vi "Spätzle_Control_myRIO.vi"(6 "error in":errorcluster) -> (0 "error out 2":errorcluster)   [LabVIEW 2014]
doc: "Mit diesem VI wird eine Autowäsche simuliert. Mit den Waschprogrammelementen wählen Sie die gewünschten Optionen aus. Wenn keine Option ausgewählt wird, ist die Hochdruckreinigung das Standardwaschprogramm. Nach Klick auf \"Start\" beginnt die Wäsche. Mit dem Element \"Schieberegler für Fahrzeugposition\" wird die Position des Fahrzeugs simuliert. Wenn sich das Fahrzeug in der falschen Position für das aktuelle Programm befindet, leuchtet die entsprechende Anzeige und das Fahrzeug muss bewegt werden. Die Anzeige der Waschanlage stellt den aktuellen Status des Waschprogramms dar. Mit der Schaltfläche \"Programm stoppen\" wird die Autowaschanlage sofort gestoppt."
uses:
  Controls/Indicators.ctl
  Controls/State Control Enum.ctl
  Controls/Conveyor Belt Functions.ctl
  <vilib>/myRIO/Instrument Drivers/Onboard IO/DIO/typedefs/DIO Reference.ctl
  <vilib>/myRIO/Common/Instrument Driver Framework/Utilities/typedefs/myRIO Generic Hardware Reference.ctl
  <vilib>/myRIO/Common/Instrument Driver Framework/Utilities/typedefs/Hardware Version Enum.ctl
  <vilib>/myRIO/Common/Instrument Driver Framework/Utilities/typedefs/myRIO v1.0 Reference.ctl
  <vilib>/myRIO/Common/Instrument Driver Framework/Utilities/typedefs/Generic FPGA Reference.ctl
  <vilib>/myRIO/Common/Instrument Driver Framework/myRIO v1.0/DIO/typedefs/DIO Channels List.ctl
  <vilib>/myRIO/Common/Instrument Driver Framework/myRIO v1.0/DIO/typedefs/DIO Channels Enum.ctl
  <vilib>/userdefined/High Color/nirio_resource_hc.ctl
  <vilib>/myRIO/Common/Instrument Driver Framework/myRIO v1.0/DIO/vis/myRIO v1.1 Open DIO.vi
  <vilib>/myRIO/Common/Instrument Driver Framework/Utilities/vis/Is FPGA Ref Available.vi
  <vilib>/myRIO/Instrument Drivers/Onboard IO/DIO/vis/Write.vi
  <vilib>/myRIO/Common/Instrument Driver Framework/Utilities/vis/Validate Channels.vi
  <vilib>/myRIO/Common/Instrument Driver Framework/myRIO v1.0/DIO/vis/myRIO v1.0 Reserve DIO.vi
  <vilib>/myRIO/Common/Instrument Driver Framework/myRIO v1.0/DIO/vis/myRIO v1.0 Close DIO.vi
  <vilib>/myRIO/Common/Instrument Driver Framework/myRIO v1.0/UART/vis/myRIO v1.0 Close UART.vi
  <vilib>/myRIO/Common/Instrument Driver Framework/myRIO v1.0/Resource Manager/vis/myRIO v1.0 Reserve Channel List.vi
  <vilib>/myRIO/Common/Instrument Driver Framework/myRIO v1.0/DIO/vis/myRIO v1.0 Build MUX Configuration DIO.vi
  <vilib>/myRIO/Common/Instrument Driver Framework/myRIO v1.0/DIO/vis/myRIO v1.0 Unreserve DIO.vi
  <vilib>/myRIO/Common/Instrument Driver Framework/myRIO v1.0/Resource Manager/vis/myRIO v1.0 Reserve Channel.vi
  <vilib>/myRIO/Common/Instrument Driver Framework/myRIO v1.0/Resource Manager/vis/myRIO v1.0 Unreserve Channel.vi
  <vilib>/myRIO/Common/Instrument Driver Framework/myRIO v1.0/Resource Manager/vis/myRIO v1.0 Create Configuration List.vi
  <vilib>/myRIO/Common/Instrument Driver Framework/myRIO v1.0/Resource Manager/vis/myRIO v1.0 Unreserve Channel List.vi
  <vilib>/myRIO/Common/Instrument Driver Framework/myRIO v1.0/Resource Manager/vis/myRIO v1.0 Build Mutex Name.vi
  <vilib>/Utility/VariantDataType/GetNumericInfo.vi
  <vilib>/Utility/error.llb/Error Cluster From Error Code.vi
  <vilib>/myRIO/Common/Instrument Driver Framework/myRIO v1.0/myRIO v1.1 Open.vi
  <vilib>/myRIO/Common/Instrument Driver Framework/Utilities/vis/IO Manager.vi
  <vilib>/myRIO/Common/Instrument Driver Framework/Utilities/vis/Configuration Manager.vi
  <vilib>/myRIO/Common/Instrument Driver Framework/myRIO v1.0/Resource Manager/vis/myRIO v1.0 Configure IO.vi
  <vilib>/myRIO/Common/Instrument Driver Framework/myRIO v1.0/myRIO v1.0 Close.vi
  <vilib>/myRIO/Common/Instrument Driver Framework/myRIO v1.0/DIO/vis/myRIO v1.0 Read DIO.vi
  <vilib>/myRIO/Common/Instrument Driver Framework/myRIO v1.0/DIO/vis/myRIO v1.0 Write DIO.vi
  <vilib>/myRIO/Common/Instrument Driver Framework/myRIO v1.0/DIO/vis/myRIO v1.0 Shutdown DIO.vi
  <vilib>/myRIO/Common/Instrument Driver Framework/Utilities/vis/FPGA Ref Manager.vi
  <vilib>/myRIO/Common/Instrument Driver Framework/myRIO v1.0/myRIO v1.0 Reset FPGA.vi
  <vilib>/myRIO/Common/Instrument Driver Framework/myRIO v1.0/IRQ/vis/myRIO v1.0 IRQ Info FGV.vi
  <vilib>/myRIO/Common/Instrument Driver Framework/myRIO v1.0/IRQ/vis/myRIO v1.0 Timer IRQ Info FGV.vi
  <vilib>/myRIO/Common/Instrument Driver Framework/myRIO v1.0/IRQ/vis/myRIO v1.0 ISR Agent.vi
  <vilib>/myRIO/Instrument Drivers/Onboard IO/DIO/vis/myRIO DIO Open.xnode
  <vilib>/myRIO/Express VI/Onboard IO/DO/DO Express VI.xnode
  <vilib>/myRIO/Instrument Drivers/Onboard IO/DIO/DIO.lvlib
  <vilib>/myRIO/Instrument Drivers/Utilities/Utilities.lvlib
panel:
  in  "stop":bool
  out "?":T1
  out "Busy":bool
  # "Machine Status"
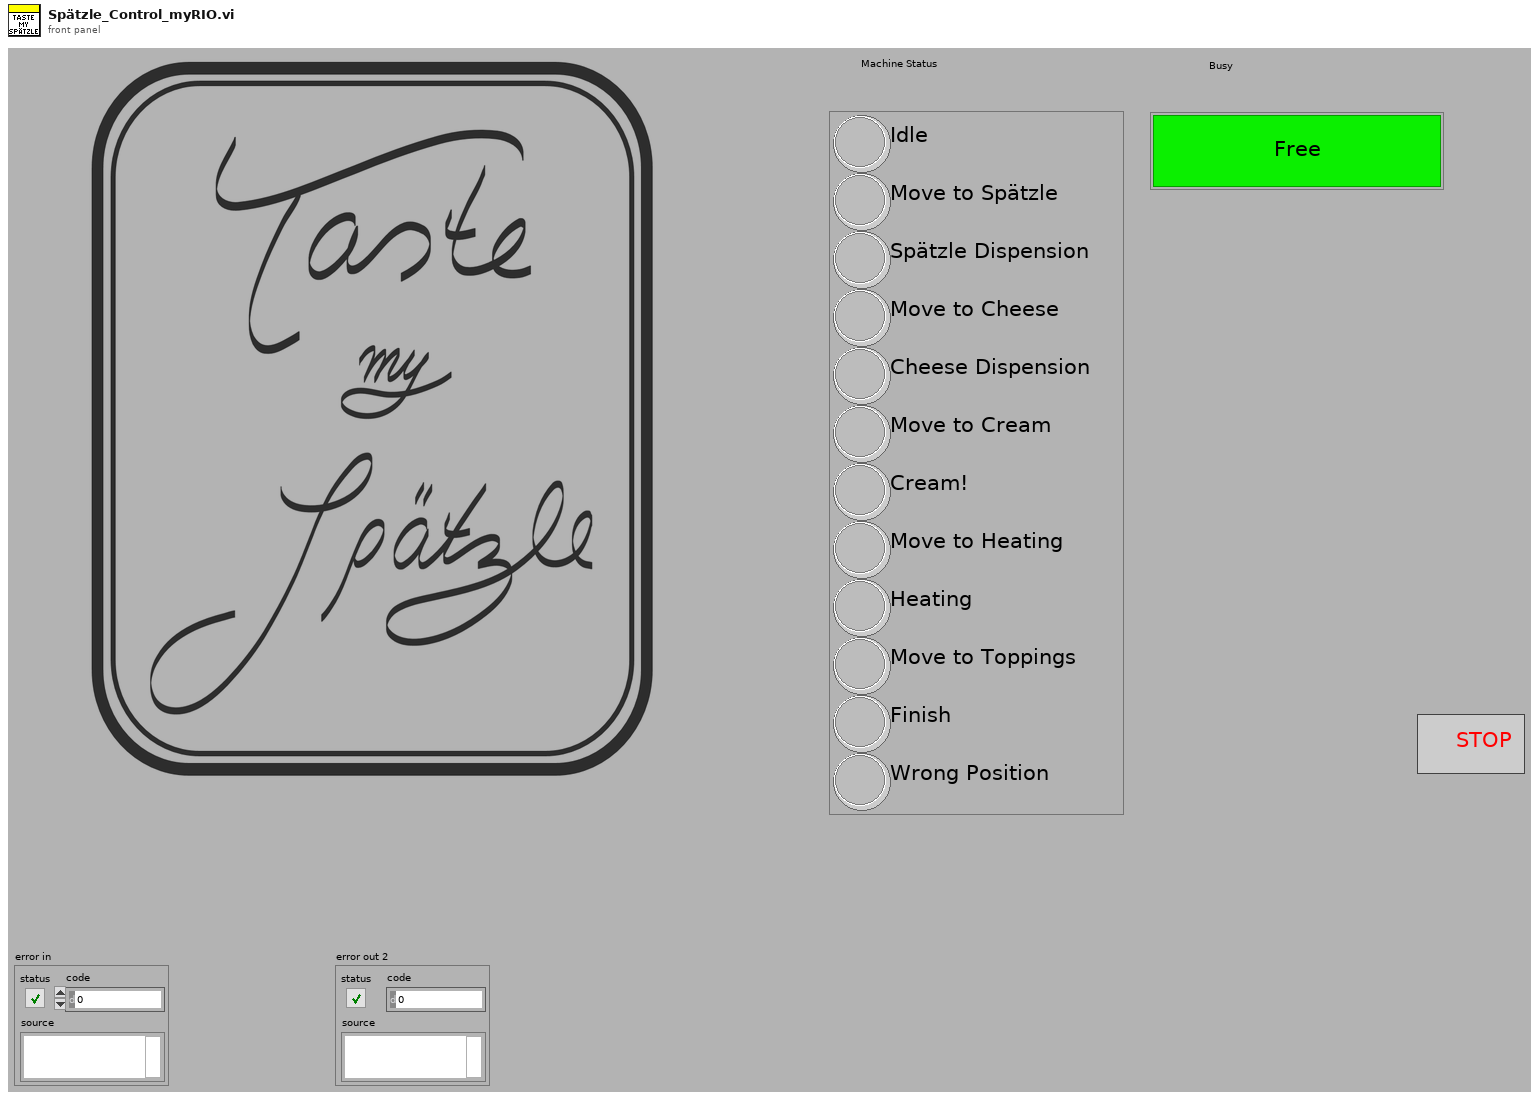
[diagram p1: front panel]
types:
  T1 = typedef "Indicators.ctl" = cluster{"Idle":bool, "Move to Spätzle":bool, "Spätzle Dispension":bool, "Move to Cheese":bool, "Cheese Dispension":bool, "Move to Cream":bool, "Cream!":bool, "Move to Heating":bool, "Heating":bool, "Move to Toppings":bool, "Finish":bool, "Wrong Position":bool}
  T2 = typedef "Conveyor Belt Functions.ctl" = enum16{"Move Forward", "Move Backward", "Stop"}
  T3 = typedef "State Control Enum.ctl" = enum16{"Initialize", "Wait for Start", "Plate Dispension", "Spätzle Dispension", "Move to Cream", "Cream", "Move to Heating", "Heating", "Cheese Dispension", "Onion Dispension", "Garlic Dispension", "Butter Dispension", "Move to Spätzle", "Move To Cheese", "Move to Exit", "Stop", "Skip"}
  T4 = typedef "DIO.lvlib/DIO Reference.ctl" = cluster{"myRIO Reference":T5, "DIO Channels List":T9}
  T5 = typedef "myRIO Generic Hardware Reference.ctl" = cluster{"myRIO Model":T6, "myRIO Hardware Reference":T7}
  T6 = typedef "Hardware Version Enum.ctl" = enum16{"Unknown", "myRIO-1900", "myRIO-1950"}
  T7 = typedef "myRIO v1.0 Reference.ctl" = cluster{"Generic FPGA Reference":T8, "Allow multiple opens":bool}
  T8 = typedef "Generic FPGA Reference.ctl" = refnum<k20>
  T9 = typedef "DIO Channels List.ctl" = T10[]
  T10 = typedef "DIO Channels Enum.ctl" = enum16{"Not Connected", "C/DIO0", "C/DIO1", "C/DIO2", "C/DIO3", "C/DIO4", "C/DIO5", "C/DIO6", "C/DIO7", "A/DIO0", "A/DIO1", "A/DIO2", "A/DIO3", "A/DIO4", "A/DIO5", "A/DIO6", "A/DIO7", "A/DIO8", "A/DIO9", "A/DIO10", "A/DIO11", "A/DIO12", "A/DIO13", "A/DIO14", "A/DIO15", "B/DIO0", "B/DIO1", "B/DIO2", "B/DIO3", "B/DIO4", "B/DIO5", "B/DIO6", "B/DIO7", "B/DIO8", "B/DIO9", "B/DIO10", "B/DIO11", "B/DIO12", "B/DIO13", "B/DIO14", "B/DIO15", "LED0", "LED1", "LED2", "LED3", "Button0"}
  T11 = typedef "nirio_resource_hc.ctl" = tag
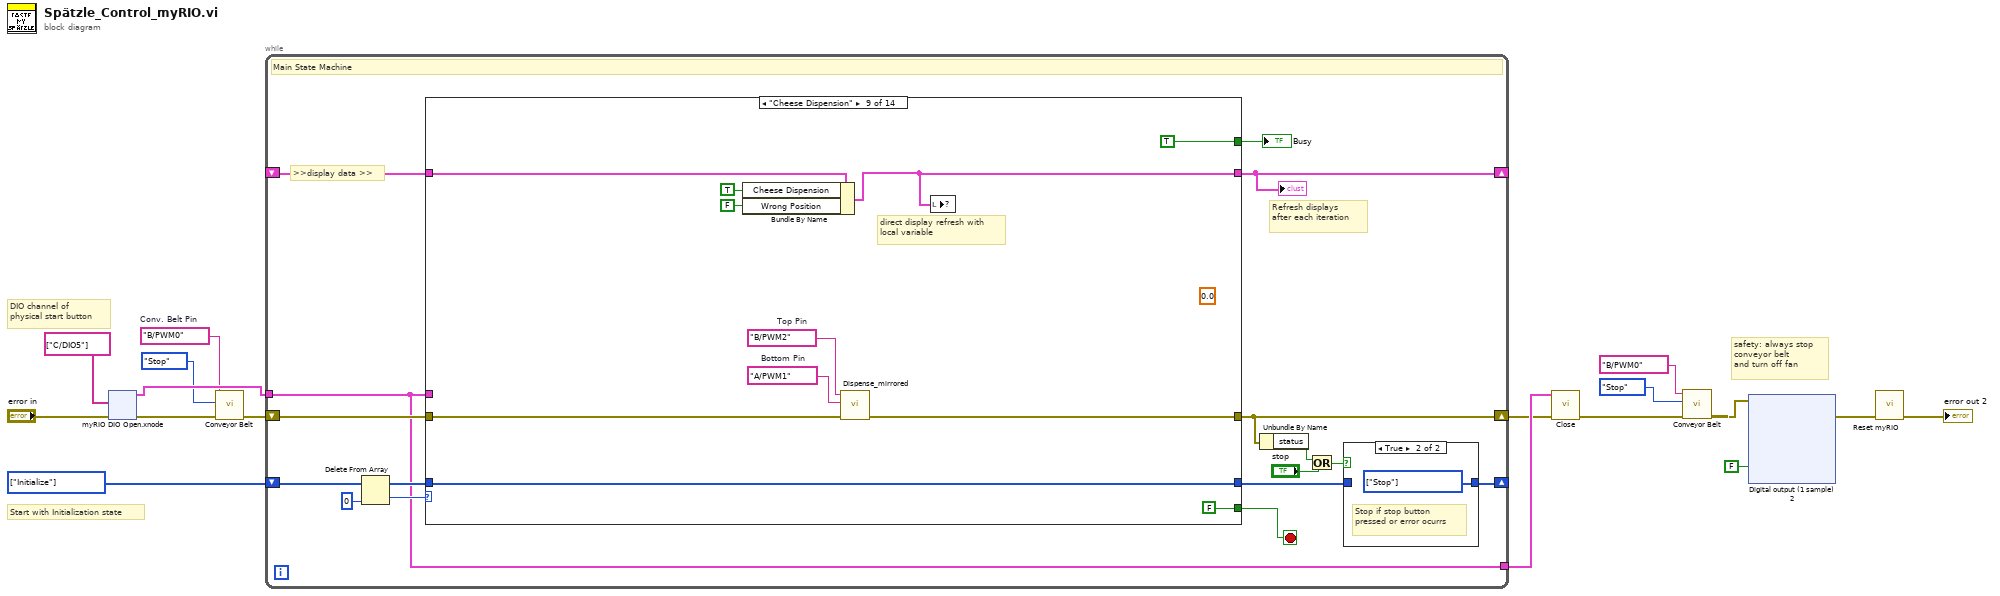
[diagram p0: block diagram]
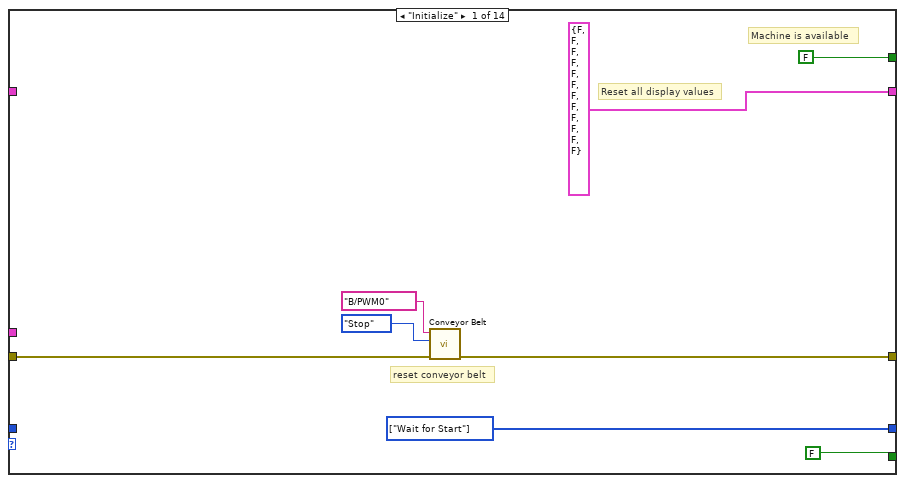
[diagram p3: hidden frame]
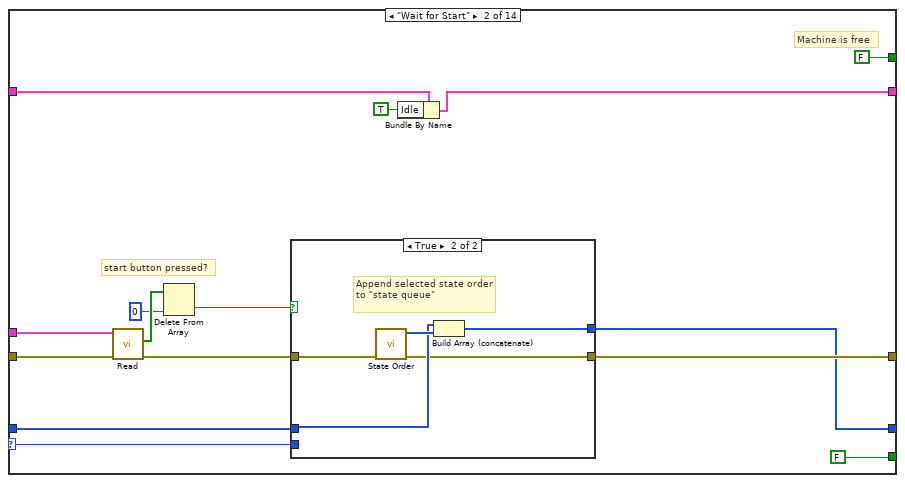
[diagram p4: hidden frame]
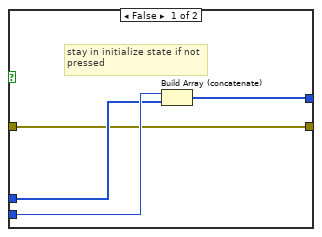
[diagram p5: hidden frame]
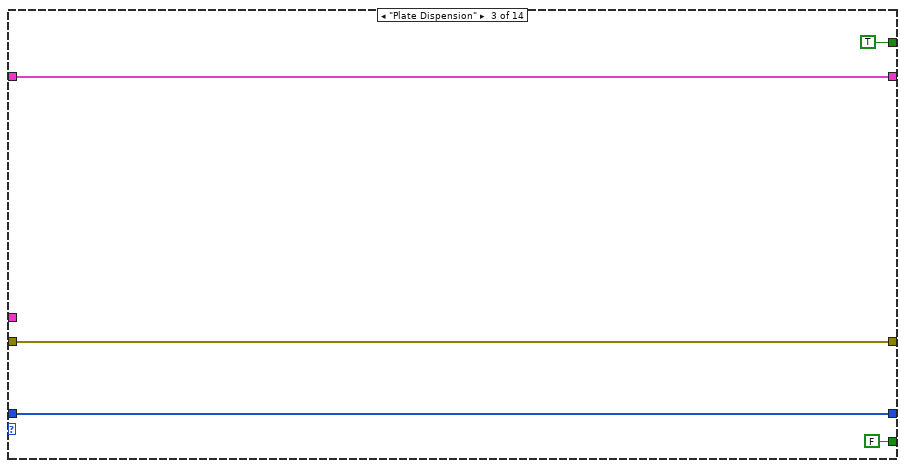
[diagram p6: hidden frame]
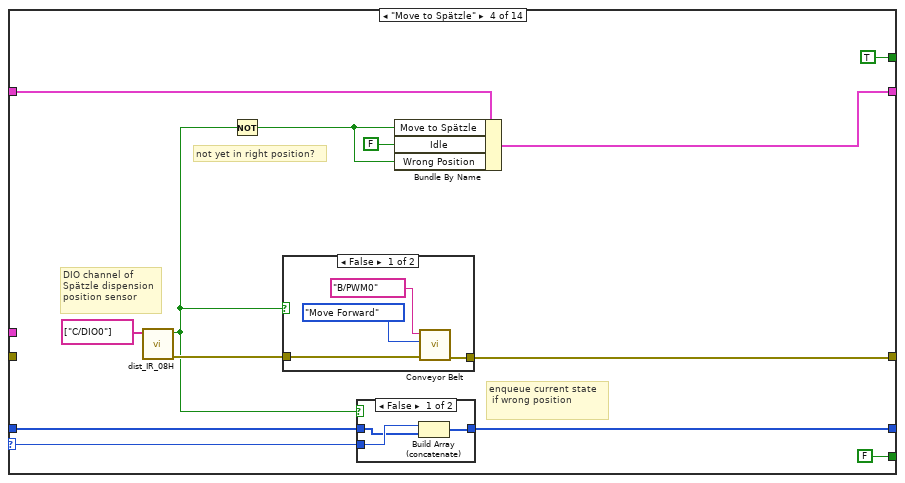
[diagram p7: hidden frame]
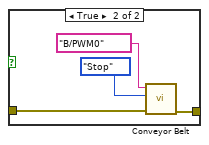
[diagram p8: hidden frame]
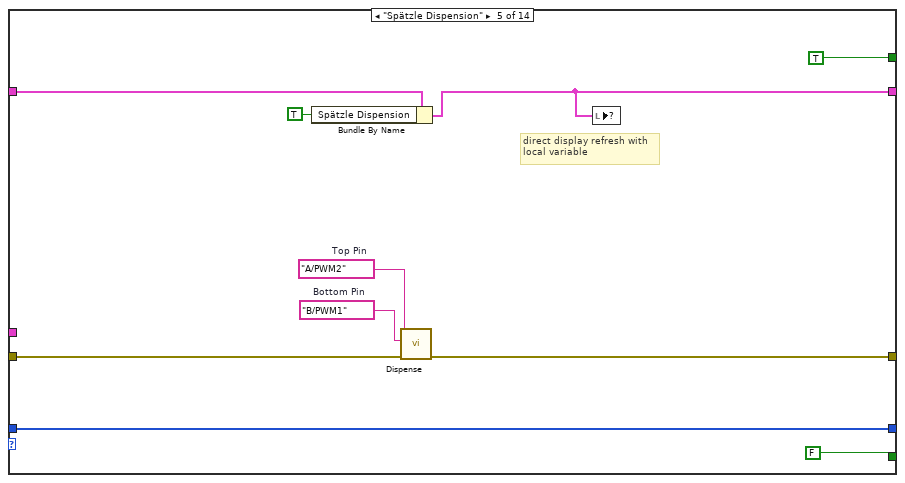
[diagram p10: hidden frame]
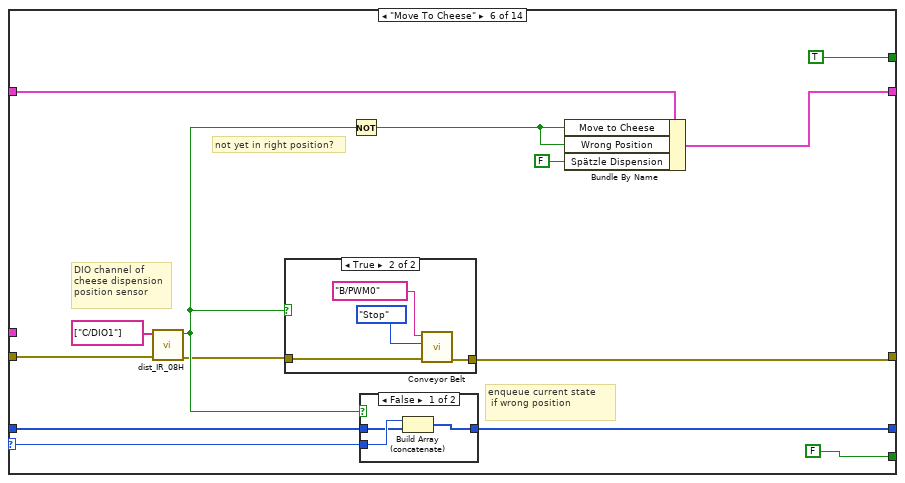
[diagram p11: hidden frame]
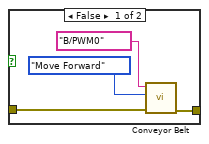
[diagram p12: hidden frame]
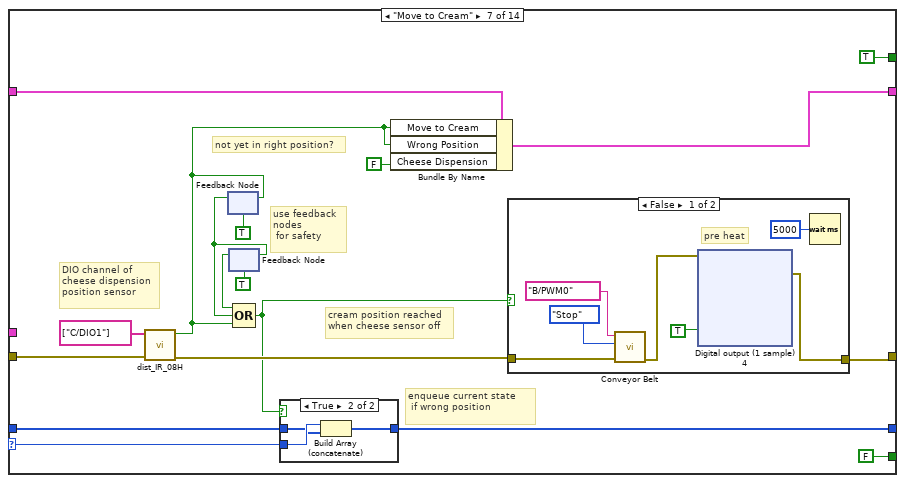
[diagram p14: hidden frame]
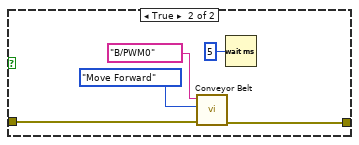
[diagram p15: hidden frame]
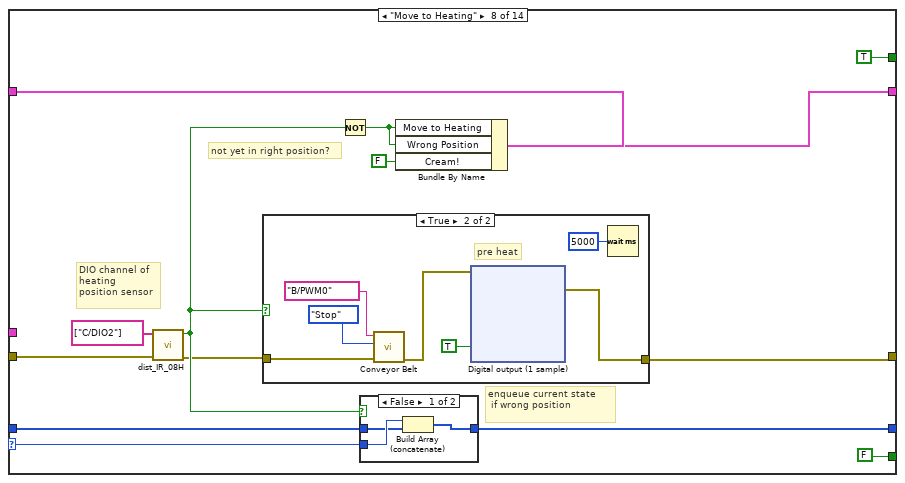
[diagram p17: hidden frame]
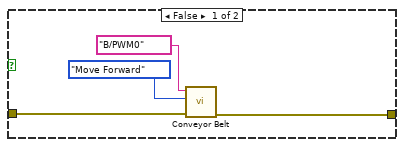
[diagram p18: hidden frame]
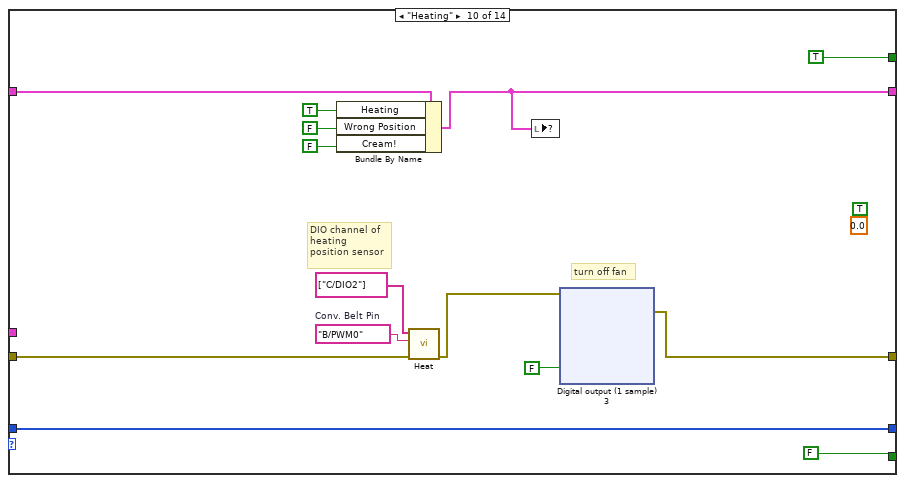
[diagram p20: hidden frame]
diagram:
  w1 = tag "B/PWM0"  # Conv. Belt Pin
  w17 = T3[] [enum."Initialize"] items=["Initialize", "Wait for Start", "Plate Dispension", "Spätzle Dispension", "Move to Cream", "Cream", "Move to Heating", "Heating", "Cheese Dispension", "Onion Dispension", "Garlic Dispension", "Butter Dispension", "Move to Spätzle", "Move To Cheese", "Move to Exit", "Stop", "Skip"]
  # "safety: always stop \nconveyor belt\nand turn off fan"
  # "DIO channel of\nphysical start button"
  # "Start with Initialization state"
  n1 = xnode "myRIO DIO Open.xnode"("error in (no error)"="error in", "Channel Names"=tag[] ["C/DIO5"]) -> ("error out"=w6:errorcluster, "DIO Ref Out"=w14:T4)  [unwired: 1 in]
  n2 = call "Conveyor Belt.vi"("error in (no error)"=w6, "Function"=Conveyor_Belt_Functions."Stop", "Conv. Belt Pin"=w1) -> ("error out"=w7:errorcluster)  [unwired: 8 in]
  n3 = while "While-Schleife" {
    shift-right: [w26] -> _
    shift-left: w17 -> [w22]
    shift-right: [w29] -> _
    shift-left: _ -> [w30]
    shift-right: [w21] -> w12
    shift-left: w7 -> [w19]
    tunnel: w14 -> [w18]
    tunnel: [w18] -> w13
    stop <- w25 stop-if-true
    # "Refresh displays after each iteration"
    # ">>display data >>"
    # "Main State Machine"
    n4 = Delete From Array ("Aus Array entfernen")(array=w22, index=0 ("Index")) -> (deleted portion=w31:T3, array with subset deleted=w32:T3[])  [unwired: 1 in]
    n5 = case "Case-Struktur" shown="\"Cheese Dispension\"" w31 {
      selector: w31 -> [_ w53 _ w79 _ w116 w146 w211 _ _ _ _ _ _]
      tunnel: w32 -> [_ w56 w70 w80 w104 w117 w147 w212 w271 w282 w330 w341 _ _]
      tunnel: [w40 w54 w70 w81 w104 w115 w145 w210 w271 w282 w330 w341 w354 w375] -> w27
      tunnel: [T1 {"Idle"=FALSE, "Move to Spätzle"=FALSE, "Spätzle Dispension"=FALSE, "Move to Cheese"=FALSE, "Cheese Dispension"=FALSE, "Move to Cream"=FALSE, "Cream!"=FALSE, "Move to Heating"=FALSE, "Heating"=FALSE, "Move to Toppings"=FALSE, "Finish"=FALSE, "Wrong Position"=FALSE} ("Anzeigen der Waschanlage 2") w51 w72 w84 w103 w120 w150 w215 w270 w280 w329 w342 w356 T1 {"Idle"=FALSE, "Move to Spätzle"=FALSE, "Spätzle Dispension"=FALSE, "Move to Cheese"=FALSE, "Cheese Dispension"=FALSE, "Move to Cream"=FALSE, "Cream!"=FALSE, "Move to Heating"=FALSE, "Heating"=FALSE, "Move to Toppings"=FALSE, "Finish"=FALSE, "Wrong Position"=FALSE} ("Anzeigen der Waschanlage 2")] -> w29
      tunnel: w30 -> [_ w52 w72 w85 w106 w121 w151 w216 w276 w290 w336 w342 w355 _]
      tunnel: [FALSE ("Einfahrt") FALSE ("Einfahrt") TRUE ("Einfahrt") TRUE ("Einfahrt") TRUE ("Einfahrt") TRUE ("Einfahrt") TRUE ("Einfahrt") TRUE ("Einfahrt") TRUE ("Einfahrt") TRUE ("Einfahrt") TRUE ("Einfahrt") TRUE ("Einfahrt") TRUE ("Einfahrt") FALSE ("Einfahrt")] -> w28
      tunnel: [FALSE ("Einfahrt") FALSE ("Einfahrt") FALSE ("Einfahrt") FALSE ("Einfahrt") FALSE ("Einfahrt") FALSE ("Einfahrt") FALSE ("Einfahrt") FALSE ("Einfahrt") FALSE ("Einfahrt") FALSE ("Einfahrt") FALSE ("Einfahrt") FALSE ("Einfahrt") FALSE ("Einfahrt") TRUE ("Einfahrt")] -> w25
      tunnel: [w39 w55 w68 w76 w98 w111 w142 w206 w274 w283 w333 w338 w347 w374] -> w21
      tunnel: w19 -> [w36 w47 w68 _ w101 w108 w134 w203 w267 w279 w327 w338 w343 w374]
      tunnel: w18 -> [_ w44 _ _ _ _ _ _ _ _ _ _ _ _]
      frame "Initialize" {
        w40 = T3[] [enum."Wait for Start"] items=["Initialize", "Wait for Start", "Plate Dispension", "Spätzle Dispension", "Move to Cream", "Cream", "Move to Heating", "Heating", "Cheese Dispension", "Onion Dispension", "Garlic Dispension", "Butter Dispension", "Move to Spätzle", "Move To Cheese", "Move to Exit", "Stop", "Skip"]
        # "reset conveyor belt"
        # "Machine is available"
        # "Reset all display values"
        n6 = call "Conveyor Belt.vi"("error in (no error)"=w36, "Function"=Conveyor_Belt_Functions."Stop", "Conv. Belt Pin"=tag "B/PWM0") -> ("error out"=w39:errorcluster)  [unwired: 8 in]
      }
      frame "Wait for Start" {
        # "start button pressed?"
        # "Machine is free"
        n7 = call <vilib>:"Read.vi"("error in (no error)"=w47, "DIO Ref In"=w44) -> ("error out"=w46:errorcluster, "Values"=w49:bool[])  [unwired: 7 in, 1 out]
        n8 = Delete From Array(array=w49, index=0) -> (deleted portion=w45:bool)  [unwired: 1 in, 1 out]
        n9 = case shown="True" w45 {
          tunnel: [w59 w64] -> w55
          tunnel: [w62 w66] -> w54
          tunnel: w56 -> [w60 w65]
          tunnel: w53 -> [w61 _]
          tunnel: w46 -> [w59 w63]
          frame False {
            # "stay in initialize state if not\npressed"
            n10 = Build Array (concatenate) ("Array erstellen")(w61, w60) -> (w62:T3[])
          }
          frame True {
            # "Append selected state order to \"state queue\""
            n11 = call "State Order.vi"("Fehler (Eingang)"=w63) -> ("Fehler (Ausgang)"=w64:errorcluster, "States"=w67:T3[])  [unwired: 1 in, 8 out]
            n12 = Build Array (concatenate) ("Array erstellen")(w65, w67) -> (w66:T3[])
          }
        }
        n13 = Bundle By Name ("Nach Namen bündeln")(cluster=w52, "Idle"=TRUE) -> (w51:T1)
      }
      frame "Plate Dispension" {
      }
      frame "Move to Spätzle" {
        # "not yet in right position?"
        # "DIO channel of\nSpätzle dispension\nposition sensor"
        # "enqueue current state\n if wrong position"
        n14 = call "dist_IR_08H.vi"("Channel Names"=tag[] ["C/DIO0"]) -> ("error out 2"=w77:errorcluster, "sensor signal (A/DIO0 (Pin 11))"=w75:bool)  [unwired: 9 in]
        n15 = Not(x=w75) -> (.not. x?=w73:bool)
        n16 = case shown="False" w75 {
          tunnel: w77 -> [w89 w93]
          tunnel: [w88 w92] -> w76
          frame False {
            n17 = call "Conveyor Belt.vi"("error in (no error)"=w89, "Function"=Conveyor_Belt_Functions."Move Forward", "Conv. Belt Pin"=tag "B/PWM0") -> ("error out"=w88:errorcluster)  [unwired: 8 in]
          }
          frame True {
            n18 = call "Conveyor Belt.vi"("error in (no error)"=w93, "Function"=Conveyor_Belt_Functions."Stop", "Conv. Belt Pin"=tag "B/PWM0") -> ("error out"=w92:errorcluster)  [unwired: 8 in]
          }
        }
        n19 = case shown="False" w75 {
          tunnel: [w94 w97] -> w81
          tunnel: w80 -> [w95 w97]
          tunnel: w79 -> [w96 _]
          frame False {
            n20 = Build Array (concatenate)(w96, w95) -> (w94:T3[])
          }
          frame True {
          }
        }
        n21 = Bundle By Name ("Nach Namen bündeln")(cluster=w85, "Move to Spätzle"=w73, "Idle"=FALSE ("Spätzle Dispension"), "Wrong Position"=w73) -> (w84:T1)
      }
      frame "Spätzle Dispension" {
        w100 = tag "B/PWM1"  # Bottom Pin
        w99 = tag "A/PWM2"  # Top Pin
        # "direct display refresh with\nlocal variable"
        n22 = Bundle By Name ("Nach Namen bündeln")(cluster=w106, "Spätzle Dispension"=TRUE) -> (w103:T1)
        n23 = call "Dispense.vi"("error in (no error)"=w101, "Bottom Pin"=w100, "Top Pin"=w99) -> ("error out"=w98:errorcluster)  [unwired: 7 in, 1 out]
        n24 = local write item#1(w103) -> ()
      }
      frame "Move To Cheese" {
        # "not yet in right position?"
        # "DIO channel of\ncheese dispension\nposition sensor"
        # "enqueue current state\n if wrong position"
        n25 = call "dist_IR_08H.vi"("error in (no error) 2"=w108, "Channel Names"=tag[] ["C/DIO1"]) -> ("error out 2"=w112:errorcluster, "sensor signal (A/DIO0 (Pin 11))"=w113:bool)  [unwired: 8 in]
        n26 = case shown="True" w113 {
          tunnel: w112 -> [w125 w129]
          tunnel: [w124 w128] -> w111
          frame False {
            n27 = call "Conveyor Belt.vi"("error in (no error)"=w125, "Function"=Conveyor_Belt_Functions."Move Forward", "Conv. Belt Pin"=tag "B/PWM0") -> ("error out"=w124:errorcluster)  [unwired: 8 in]
          }
          frame True {
            n28 = call "Conveyor Belt.vi"("error in (no error)"=w129, "Function"=Conveyor_Belt_Functions."Stop", "Conv. Belt Pin"=tag "B/PWM0") -> ("error out"=w128:errorcluster)  [unwired: 8 in]
          }
        }
        n29 = Not(x=w113) -> (.not. x?=w110:bool)
        n30 = case shown="False" w113 {
          tunnel: [w132 w133] -> w115
          tunnel: w116 -> [w131 _]
          tunnel: w117 -> [w130 w133]
          frame False {
            n31 = Build Array (concatenate) ("Array erstellen")(w131, w130) -> (w132:T3[])
          }
          frame True {
          }
        }
        n32 = Bundle By Name ("Nach Namen bündeln")(cluster=w121, "Move to Cheese"=w110, "Wrong Position"=w110, "Spätzle Dispension"=FALSE) -> (w120:T1)
      }
      frame "Move to Cream" {
        # "cream position reached\nwhen cheese sensor off"
        # "use feedback \nnodes\n for safety"
        # "not yet in right position?"
        # "DIO channel of\ncheese dispension\nposition sensor"
        # "enqueue current state\n if wrong position"
        n33 = call "dist_IR_08H.vi"("error in (no error) 2"=w134, "Channel Names"=tag[] ["C/DIO1"]) -> ("error out 2"=w143:errorcluster, "sensor signal (A/DIO0 (Pin 11))"=w135:bool)  [unwired: 8 in]
        n34 = feedback-in #1(w135) -> ()
        n35 = feedback #1(TRUE ("sensor signal (A/DIO0 (Pin 11))")) -> (w140:bool)
        n36 = feedback-in #2(w140) -> ()
        n37 = feedback #2(TRUE ("sensor signal (A/DIO0 (Pin 11))")) -> (w138:bool)
        n38 = Compound Arithmetic op=OR(w138, w140, w135) -> (w137:bool)
        n39 = case shown="True" w137 {
          tunnel: [w199 w202] -> w145
          tunnel: w146 -> [_ w201]
          tunnel: w147 -> [w199 w200]
          frame False {
          }
          frame True {
            n40 = Build Array (concatenate) ("Array erstellen")(w201, w200) -> (w202:T3[])
          }
        }
        n41 = Bundle By Name ("Nach Namen bündeln")(cluster=w151, "Move to Cream"=w135, "Wrong Position"=w135, "Cheese Dispension"=FALSE) -> (w150:T1)
        n42 = case shown="False" w137 {
          tunnel: w143 -> [w158 w198]
          tunnel: [w153 w197] -> w142
          frame False {
            # "pre heat"
            n43 = call "Conveyor Belt.vi"("error in (no error)"=w158, "Function"=Conveyor_Belt_Functions."Stop", "Conv. Belt Pin"=tag "B/PWM0") -> ("error out"=w152:errorcluster)  [unwired: 8 in]
            n44 = xnode "Digital output (1 sample) 4"("C/DIO4 (DIO4)"=TRUE, "error in (no error)"=w152) -> ("error out"=w153:errorcluster)
            n45 = Wait (ms) ("Warten (ms)")(milliseconds to wait=u32 5000 ("Zu wartende ms")) -> ()  [unwired: 1 out]
          }
          frame True {
            n46 = call "Conveyor Belt.vi"("error in (no error)"=w198, "Function"=Conveyor_Belt_Functions."Move Forward", "Conv. Belt Pin"=tag "B/PWM0") -> ("error out"=w197:errorcluster)  [unwired: 8 in]
            n47 = Wait (ms)(milliseconds to wait=u32 5) -> ()  [unwired: 1 out]
          }
        }
      }
      frame "Move to Heating" {
        # "not yet in right position?"
        # "DIO channel of\nheating\nposition sensor"
        # "enqueue current state\n if wrong position"
        n48 = call "dist_IR_08H.vi"("error in (no error) 2"=w203, "Channel Names"=tag[] ["C/DIO2"]) -> ("error out 2"=w207:errorcluster, "sensor signal (A/DIO0 (Pin 11))"=w208:bool)  [unwired: 8 in]
        n49 = case shown="True" w208 {
          tunnel: w207 -> [w220 w227]
          tunnel: [w219 w223] -> w206
          frame False {
            n50 = call "Conveyor Belt.vi"("error in (no error)"=w220, "Function"=Conveyor_Belt_Functions."Move Forward", "Conv. Belt Pin"=tag "B/PWM0") -> ("error out"=w219:errorcluster)  [unwired: 8 in]
          }
          frame True {
            # "pre heat"
            n51 = call "Conveyor Belt.vi"("error in (no error)"=w227, "Function"=Conveyor_Belt_Functions."Stop", "Conv. Belt Pin"=tag "B/PWM0") -> ("error out"=w224:errorcluster)  [unwired: 8 in]
            n52 = xnode "Digital output (1 sample)"("C/DIO4 (DIO4)"=TRUE, "error in (no error)"=w224) -> ("error out"=w223:errorcluster)
            n53 = Wait (ms) ("Warten (ms)")(milliseconds to wait=u32 5000 ("Zu wartende ms")) -> ()  [unwired: 1 out]
          }
        }
        n54 = Not(x=w208) -> (.not. x?=w205:bool)
        n55 = case shown="False" w208 {
          tunnel: [w265 w266] -> w210
          tunnel: w211 -> [w264 _]
          tunnel: w212 -> [w263 w266]
          frame False {
            n56 = Build Array (concatenate) ("Array erstellen")(w264, w263) -> (w265:T3[])
          }
          frame True {
          }
        }
        n57 = Bundle By Name ("Nach Namen bündeln")(cluster=w216, "Move to Heating"=w205, "Wrong Position"=w205, "Cream!"=FALSE ("Wrong Position")) -> (w215:T1)
      }
      frame "Cheese Dispension" {
        w272 = tag "A/PWM1"  # Bottom Pin
        w273 = tag "B/PWM2"  # Top Pin
        (unwired) 0.0 ("Verstrichene Zeit")
        # "direct display refresh with\nlocal variable"
        n58 = Bundle By Name ("Nach Namen bündeln")(cluster=w276, "Cheese Dispension"=TRUE, "Wrong Position"=FALSE) -> (w270:T1)
        n59 = call "Dispense_mirrored.vi"("error in (no error)"=w267, "Bottom Pin"=w272, "Top Pin"=w273) -> ("error out"=w274:errorcluster)  [unwired: 7 in, 1 out]
        n60 = local write item#1(w270) -> ()
      }
      frame "Heating" {
        w287 = tag "B/PWM0"  # Conv. Belt Pin
        (unwired) 0.0 ("Verstrichene Zeit")
        (unwired) TRUE ("Zeit abgelaufen?")
        # "turn off fan"
        # "DIO channel of\nheating\nposition sensor"
        n61 = Bundle By Name ("Nach Namen bündeln")(cluster=w290, "Heating"=TRUE, "Wrong Position"=FALSE, "Cream!"=FALSE ("Wrong Position")) -> (w280:T1)
        n62 = call "Heat.vi"("error in (no error)"=w279, "Conv. Belt Pin"=w287, "Heat Position Sensor"=tag[] ["C/DIO2"] ("Channel Names")) -> ("error out 2"=w284:errorcluster)  [unwired: 8 in]
        n63 = local write item#1(w280) -> ()
        n64 = xnode "Digital output (1 sample) 3"("C/DIO4 (DIO4)"=FALSE, "error in (no error)"=w284) -> ("error out"=w283:errorcluster)
      }
      frame "Cream" {
        w331 = tag "B/PWM0"  # Conv. Belt Pin
        w332 = tag "A/PWM0"  # Cream Servo Pin
        n65 = Bundle By Name ("Nach Namen bündeln")(cluster=w336, "Cream!"=TRUE ("Heating"), "Move to Cream"=FALSE) -> (w329:T1)
        n66 = call "Cream.vi"("error in (no error)"=w327, "Servo Pin"=w332, "Conv. Belt Pin"=w331) -> ("error out 2"=w333:errorcluster)  [unwired: 8 in]
        n67 = local write item#1(w329) -> ()
      }
      frame "Skip", Default {
      }
      frame "Move to Exit" {
        # "DIO channel of\nexit\nposition sensor"
        n68 = call "dist_IR_08H.vi"("error in (no error) 2"=w343, "Channel Names"=tag[] ["C/DIO3"]) -> ("error out 2"=w352:errorcluster, "sensor signal (A/DIO0 (Pin 11))"=w346:bool)  [unwired: 8 in]
        n69 = case shown="True" w346 {
          tunnel: w352 -> [w360 w361]
          tunnel: [w359 w363] -> w348
          frame False {
            n70 = call "Conveyor Belt.vi"("error in (no error)"=w360, "Function"=Conveyor_Belt_Functions."Move Forward", "Conv. Belt Pin"=tag "B/PWM0") -> ("error out"=w359:errorcluster)  [unwired: 8 in]
          }
          frame True {
            # "small delay to come to right position for robot"
            n71 = flat-sequence {
              tunnel: w361 -> [w365]
              tunnel: [w365] -> w362
              tunnel: [w369] -> w363
              tunnel: w362 -> [w366]
              frame #0 {
                n72 = Wait (ms)(milliseconds to wait=u32 500) -> ()  [unwired: 1 out]
              }
              frame #1 {
                n73 = call "Conveyor Belt.vi"("error in (no error)"=w366, "Function"=Conveyor_Belt_Functions."Stop", "Conv. Belt Pin"=tag "B/PWM0") -> ("error out"=w369:errorcluster)  [unwired: 8 in]
              }
            }
          }
        }
        n74 = Not(x=w346) -> (.not. x?=w351:bool)
        n75 = Not(x=w346) -> (.not. x?=w350:bool)
        n76 = Bundle By Name ("Nach Namen bündeln")(cluster=w355, "Move to Toppings"=w350, "Wrong Position"=w351, "Heating"=FALSE ("Wrong Position")) -> (w356:T1)
        n77 = case shown="False" w346 {
          tunnel: [w371 w373] -> w354
          tunnel: w348 -> [w370 w372]
          tunnel: [w370 w372] -> w347
          frame False {
            w371 = T3[] [enum."Move to Exit"] items=["Initialize", "Wait for Start", "Plate Dispension", "Spätzle Dispension", "Move to Cream", "Cream", "Move to Heating", "Heating", "Cheese Dispension", "Onion Dispension", "Garlic Dispension", "Butter Dispension", "Move to Spätzle", "Move To Cheese", "Move to Exit", "Stop", "Skip"]
          }
          frame True {
            w373 = T3[] [enum."Initialize"] items=["Initialize", "Wait for Start", "Plate Dispension", "Spätzle Dispension", "Move to Cream", "Cream", "Move to Heating", "Heating", "Cheese Dispension", "Onion Dispension", "Garlic Dispension", "Butter Dispension", "Move to Spätzle", "Move To Cheese", "Move to Exit", "Stop", "Skip"]
          }
        }
      }
      frame "Stop" {
        w375 = T3[] [enum."Stop"] items=["Initialize", "Wait for Start", "Plate Dispension", "Spätzle Dispension", "Move to Cream", "Cream", "Move to Heating", "Heating", "Cheese Dispension", "Onion Dispension", "Garlic Dispension", "Butter Dispension", "Move to Spätzle", "Move To Cheese", "Move to Exit", "Stop", "Skip"]
        # "reset displays"
      }
    }
    "?" <- w29
    "Busy" <- w28
    n78 = Unbundle By Name ("Nach Namen aufschlüsseln")(w21) -> ("status"=w24:bool)
    n79 = Or ("ODER")(x=w24, y="stop") -> (x .or. y?=w23:bool)
    n80 = case "Case-Struktur" shown="True" w23 {
      tunnel: w27 -> [w34 _]
      tunnel: [w34 w35] -> w26
      frame False {
      }
      frame True {
        w35 = T3[] [enum."Stop"] items=["Initialize", "Wait for Start", "Plate Dispension", "Spätzle Dispension", "Move to Cream", "Cream", "Move to Heating", "Heating", "Cheese Dispension", "Onion Dispension", "Garlic Dispension", "Butter Dispension", "Move to Spätzle", "Move To Cheese", "Move to Exit", "Stop", "Skip"]
        # "Stop if stop button pressed or error ocurrs"
      }
    }
  }
  n81 = call "Conveyor Belt.vi"("error in (no error)"=w12, "Function"=Conveyor_Belt_Functions."Stop", "Conv. Belt Pin"=tag "B/PWM0") -> ("error out"=w11:errorcluster)  [unwired: 8 in]
  n82 = call <vilib>:"Close.vi"("error in (no error)"=w11, "DIO Ref In"=w13) -> ("error out"=w3:errorcluster)  [unwired: 9 in]
  n83 = xnode "Digital output (1 sample) 2"("C/DIO4 (DIO4)"=FALSE, "error in (no error)"=w3) -> ("error out"=w2:errorcluster)
  n84 = call <vilib>:"Reset myRIO.vi"("error in (no error)"=w2) -> ("error out"=→"error out 2":errorcluster)  [unwired: 10 in]
